vi "SAC-Process Frame.vi"(0 "Cal.Data In":T1, 7 "AI Waveforms":dbl[][](array[numeric]), 9 "First":bool, 11 "error in (no error)":errorcluster) -> (4 "Cal.Data Out":T1, 13 "Status":string, 14 "Finished":bool, 15 "error out":errorcluster)   [LabVIEW 2020]
uses:
  Typedefs/SAC-Runtime Data.ctl
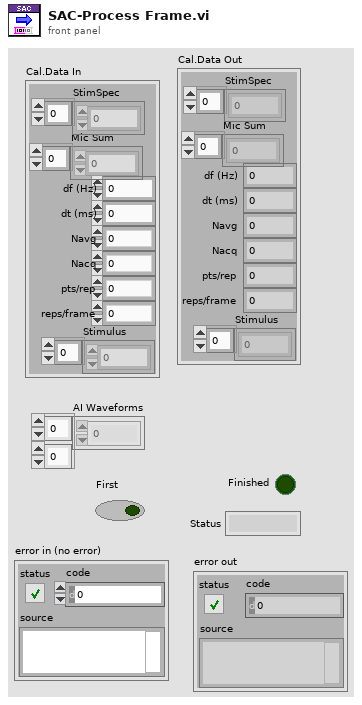
[diagram p1: front panel]
types:
  T1 = typedef "SAC-Runtime Data.ctl" = cluster{"StimSpec":cdb[], "Mic Sum":dbl[], "df (Hz)":dbl, "dt (ms)":dbl, "Navg":i32, "Nacq":i32, "pts/rep":i32, "reps/frame":i32, "Stimulus":dbl[]}
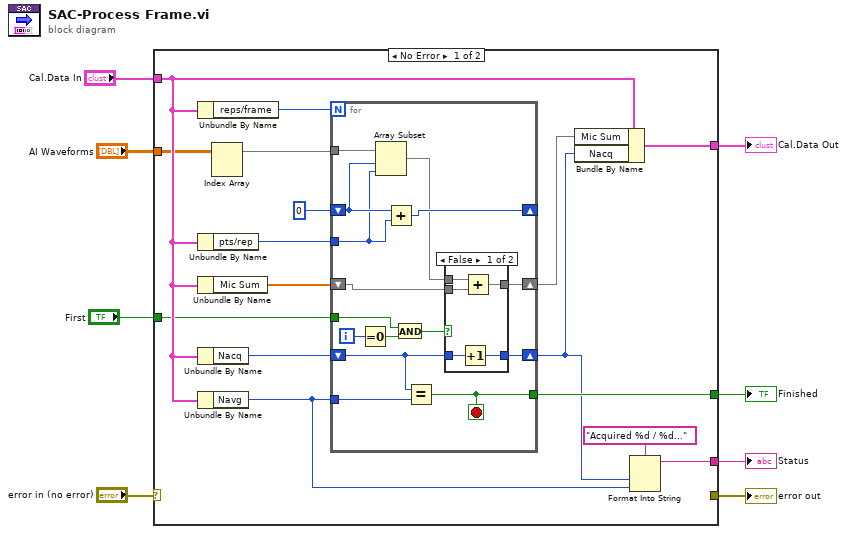
[diagram p0: block diagram]
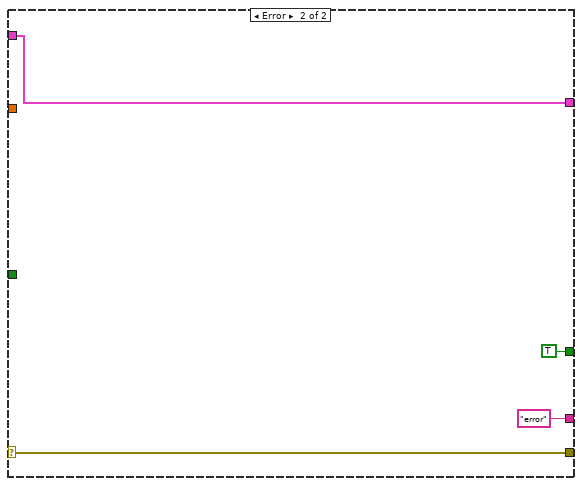
[diagram p3: hidden frame]
diagram:
  n1 = case shown="No Error" "error in (no error)" {
    selector: "error in (no error)" -> [_ w49]
    tunnel: "Cal.Data In" -> [w19 w50]
    tunnel: [w18 TRUE] -> w7
    tunnel: [w16 w50] -> w6
    tunnel: [_ w49] -> w4
    tunnel: [w14 "error"] -> w3
    tunnel: "AI Waveforms" -> [w11 _]
    tunnel: "First" -> [w10 _]
    frame No Error {
      n2 = Unbundle By Name(w19) -> ("reps/frame"=w23:i32)
      n3 = Unbundle By Name(w19) -> ("pts/rep"=w21:i32)
      n4 = Unbundle By Name(w19) -> ("Mic Sum"=w24:dbl[])
      n5 = Unbundle By Name(w19) -> ("Nacq"=w20:i32)
      n6 = Unbundle By Name(w19) -> ("Navg"=w12:i32)
      n7 = Index Array(array=w11) -> (element=w9:dbl[])  [unwired: 2 in]
      n8 = for {
        N: w23 -> [_]
        shift-right: [w36] -> w17
        shift-left: w24 -> [w37]
        tunnel: w9 -> [w39]
        shift-right: [w38] -> _
        shift-left: 0 -> [w26]
        tunnel: w21 -> [w25]
        shift-right: [w28] -> w13
        shift-left: w20 -> [w27]
        tunnel: w12 -> [w34]
        tunnel: [w33] -> w18
        tunnel: w10 -> [w30]
        i -> [w32]
        stop <- w33 stop-if-true
        n9 = Equal To 0?(x=w32) -> (x = 0?=w31:bool)
        n10 = Array Subset(array=w39, index=w26, length=w25) -> (w35:dbl[])
        n11 = Add(x=w26, y=w25) -> (x+y=w38:i32)
        n12 = And(x=w30, y=w31) -> (x .and. y?=w29:bool)
        n13 = Equal?(x=w27, y=w34) -> (x = y?=w33:bool)
        n14 = case shown="False" w29 {
          tunnel: w37 -> [w44 w46]
          tunnel: [w43 w46] -> w36
          tunnel: w35 -> [w42 _]
          tunnel: w27 -> [w41 w45]
          tunnel: [w40 w45] -> w28
          frame False {
            n15 = Increment(x=w41) -> (x+1=w40:i32)
            n16 = Add(x=w42, y=w44) -> (x+y=w43:dbl[])
          }
          frame True {
          }
        }
      }
      n17 = Bundle By Name(cluster=w19, "Mic Sum"=w17, "Nacq"=w13) -> (w16:T1)
      n18 = Format Into String(format string="Acquired %d / %d...", w13, w12) -> (resulting string=w14:string)  [unwired: 2 in, 1 out]
    }
    frame Error {
    }
  }
  "Cal.Data Out" <- w6
  "error out" <- w4
  "Status" <- w3
  "Finished" <- w7
